vi "Load dynam called VIs.vi"   [LabVIEW 2017]
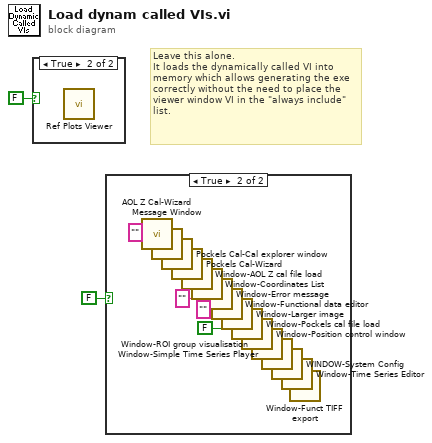
[diagram p0: block diagram]
diagram:
  # "Leave this alone.\nIt loads the dynamically called VI into memory which allows generating the exe correctly without the need to place the viewer window VI in the \"always include\" list."
  n1 = case shown="True" FALSE {
    frame False {
    }
    frame True {
      n2 = call "Ref Plots Viewer.vi"() -> ()  [unwired: 12 in]
    }
  }
  n3 = case shown="True" FALSE {
    frame False {
    }
    frame True {
      n4 = call "AOL Z Cal-Wizard.vi"() -> ()  [unwired: 12 in]
      n5 = call "Message Window.vi"("Message string"="") -> ()  [unwired: 10 in, 1 out]
      n6 = call "Pockels Cal-Cal explorer window.vi"() -> ()  [unwired: 12 in]
      n7 = call "Pockels Cal-Wizard.vi"() -> ()  [unwired: 12 in]
      n8 = call "Window-AOL Z cal file load.vi"() -> ()  [unwired: 12 in]
      n9 = call "Window-Coordinates List.vi"() -> ()  [unwired: 12 in]
      n10 = call "Window-Error message.vi"("Message"="") -> ()  [unwired: 10 in, 1 out]
      n11 = call "Window-Functional data editor.vi"() -> ()  [unwired: 12 in]
      n12 = call "Window-Larger image.vi"("Image name"="", "Open maximised"=FALSE) -> ()  [unwired: 10 in]
      n13 = call "Window-Pockels cal file load.vi"() -> ()  [unwired: 12 in]
      n14 = call "Window-Position control window.vi"() -> ()  [unwired: 12 in]
      n15 = call "Window-ROI group visualisation.vi"() -> ()  [unwired: 11 in, 1 out]
      n16 = call "Window-Simple Time Series Player.vi"() -> ()  [unwired: 12 in]
      n17 = call "WINDOW-System Config.vi"() -> ()  [unwired: 12 in]
      n18 = call "Window-Time Series Editor.vi"() -> ()  [unwired: 12 in]
      n19 = call "Window-Funct TIFF export.vi"() -> ()  [unwired: 12 in]
    }
  }
